vi "Log error.vi"(8 "error in (no error)":errorcluster, 11 "Channel in":refnum<class "Channel.lvclass">) -> (0 "error out":errorcluster, 3 "Channel out":refnum<class "Channel.lvclass">)   [LabVIEW 2018, in "Channel.lvclass"]
uses:
  Channel.lvclass
  Channel.lvclass/Channel.ctl
  State Machine/State Machine.lvclass
  Simulated_CCD_Camera/Simulated_CCD_Camera.lvclass
  <vilib>/CPE Systems NZ Ltd/Error Logger/Error Logger.lvlib
  RxTx/RxTx.lvclass
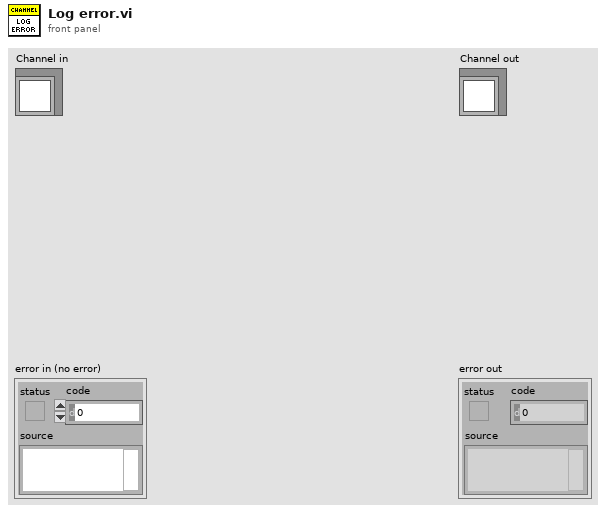
[diagram p1: front panel]
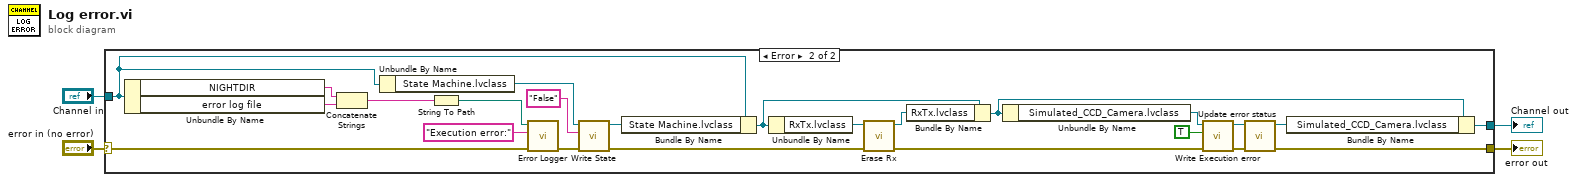
[diagram p0: block diagram]
diagram:
  n1 = case shown="Error" "error in (no error)" {
    selector: "error in (no error)" -> [w6 w27]
    tunnel: [w6 w11] -> w3
    tunnel: [w5 w15] -> w2
    tunnel: "Channel in" -> [w5 w22]
    frame No Error {
    }
    frame Error {
      n2 = Unbundle By Name(w22) -> ("NIGHTDIR"=w23:string, "error log file"=w7:string)
      n3 = Concatenate Strings(w23, w7) -> (w24:string)
      n4 = Unbundle By Name(w22) -> ("State Machine.lvclass"=w25:refnum<class "State Machine.lvclass">)
      n5 = String To Path(string=w24) -> (path=w21:path)
      n6 = call <vilib>:"Error Logger.vi"("Error To Log"=w27, "Error Label"="Execution error:", "Custom File Path"=w21) -> ("Error Out"=w26:errorcluster)  [unwired: 7 in, 1 out]
      n7 = call-dynamic "Write State.vi"("error in (no error)"=w26, "State"="False", "State Machine in"=w25) -> ("error out"=w19:errorcluster, "State Machine out"=w30:refnum<class "State Machine.lvclass">)  [unwired: 7 in]
      n8 = Bundle By Name(cluster=w22, "State Machine.lvclass"=w30) -> (w18:refnum<class "Channel.lvclass">)
      n9 = Unbundle By Name(w18) -> ("RxTx.lvclass"=w20:refnum<class "RxTx.lvclass">)
      n10 = call "Erase Rx.vi"("error in (no error)"=w19, "RxTx in"=w20) -> ("error out"=w10:errorcluster, "RxTx out"=w17:refnum<class "RxTx.lvclass">)  [unwired: 8 in]
      n11 = Bundle By Name(cluster=w18, "RxTx.lvclass"=w17) -> (w16:refnum<class "Channel.lvclass">)
      n12 = Unbundle By Name(w16) -> ("Simulated_CCD_Camera.lvclass"=w14:refnum<class "Simulated_CCD_Camera.lvclass">)
      n13 = call-dynamic "Write Execution error.vi"("error in (no error)"=w10, "Execution error"=TRUE, "Simulated_CCD_Camera in"=w14) -> ("error out"=w9:errorcluster, "Simulated_CCD_Camera out"=w13:refnum<class "Simulated_CCD_Camera.lvclass">)  [unwired: 7 in]
      n14 = call "Update error status.vi"("error in (no error)"=w9, "Simulated_CCD_Camera in"=w13) -> ("error out"=w11:errorcluster, "Simulated_CCD_Camera out"=w12:refnum<class "Simulated_CCD_Camera.lvclass">)  [unwired: 8 in]
      n15 = Bundle By Name(cluster=w16, "Simulated_CCD_Camera.lvclass"=w12) -> (w15:refnum<class "Channel.lvclass">)
    }
  }
  "error out" <- w3
  "Channel out" <- w2
